vi "Test Customer Order Sent to Handler on Submit Order.vi"(8 "error in (no error)":errorcluster, 11 "Customer Test in":refnum<class "Customer Test.lvclass">=refnum) -> (0 "error out":errorcluster, 3 "Customer Test out":refnum<class "Customer Test.lvclass">)   [LabVIEW 2020, in "Customer Test.lvclass"]
uses:
  Customer Test.lvclass
  Processes/People/Customers/Customer/Customer.lvclass
  <vilib>/Astemes/Triarc Framework/Process/Process.lvclass
  Support/Beverages/TypeDefs/Options.ctl
  Support/Beverages/Beverage/Beverage.lvclass
  Support/Beverages/TypeDefs/Drink Type.ctl
  Test Doubles/Mock Job Handler/Mock Job Handler.lvclass
  C:/git/astemes-triarc-examples/source/Coffee Shop/Processes/People/Person/Person.lvclass
  C:/Program Files (x86)/National Instruments/LabVIEW 2020/vi.lib/Astemes/Triarc Framework/View/View.lvclass
  C:/Program Files (x86)/National Instruments/LabVIEW 2020/vi.lib/Astemes/Triarc Framework/Process/Process.lvclass
  C:/Program Files (x86)/National Instruments/LabVIEW 2020/vi.lib/Astemes/Triarc Framework/Base/Base.lvclass
  C:/Program Files (x86)/National Instruments/LabVIEW 2020/vi.lib/Astemes/Triarc Framework/Error Handler Interface/Error Handler Interface.lvclass
  C:/Program Files (x86)/National Instruments/LabVIEW 2020/vi.lib/Astemes/Triarc Framework/Logging/Logging.lvclass
  C:/git/astemes-triarc-examples/source/Coffee Shop/Processes/People/Customers/Customer/Customer.lvclass
  C:/git/astemes-triarc-examples/source/Coffee Shop/Processes/People/Process Job/Job Handler.lvclass
  C:/Program Files (x86)/National Instruments/LabVIEW 2020/vi.lib/Astemes/Triarc Framework/Async Handler/Async Handler.lvclass
  <vilib>/Astemes/LUnit/Test Case.lvclass
  C:/Program Files (x86)/National Instruments/LabVIEW 2020/vi.lib/Astemes/LUnit/Test Case.lvclass
  C:/Program Files (x86)/National Instruments/LabVIEW 2020/vi.lib/Astemes/LUnit/LUnit Runnable.lvclass
  C:/git/astemes-triarc-examples/source/Coffee Shop/Tests/Test Doubles/Mock Job Handler/Mock Job Handler.lvclass
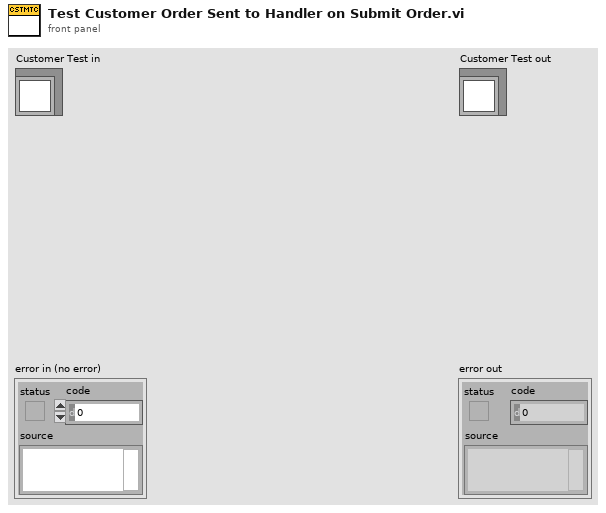
[diagram p1: front panel]
types:
  T1 = typedef "Beverage.lvclass/Drink Type.ctl" = enum16{"Dark Roast", "Decaf", "Espresso", "House Blend"}
  T2 = typedef "Beverage.lvclass/Options.ctl" = enum16{"<None>", "Milk", "Mocha", "Soy", "Whip"}
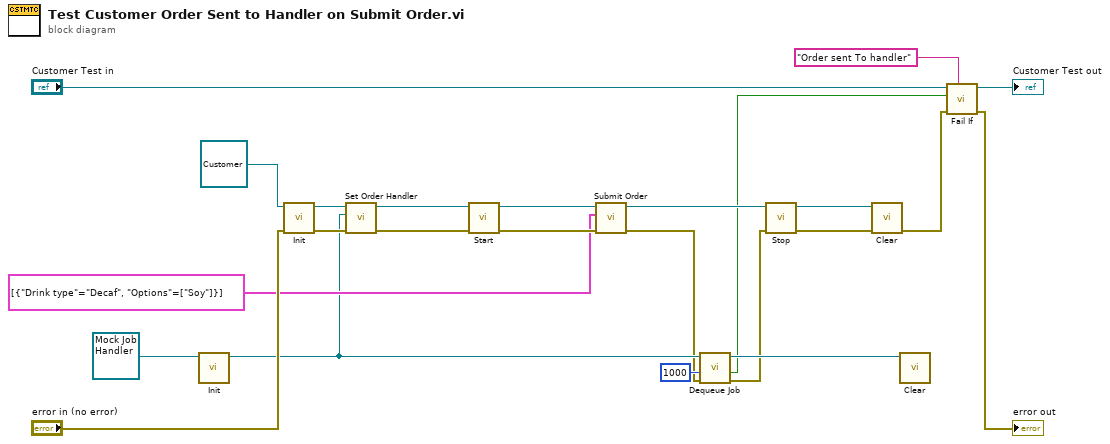
[diagram p0: block diagram]
diagram:
  n1 = call-dynamic "Init.vi"("Mock Job Handler In"=refnum<class "Mock Job Handler.lvclass"> refnum ("Mock Job Handler.lvclass")) -> ("Mock Job Handler Out"=w5:refnum<class "Mock Job Handler.lvclass">)  [unwired: 9 in, 1 out]
  n2 = call-dynamic "Init.vi"("error in (no error)"="error in (no error)", "View In"=refnum<class "Customer.lvclass"> refnum ("Customer.lvclass")) -> ("error out"=w23:errorcluster, "View Out"=w9:refnum<class "Customer.lvclass">)  [unwired: 8 in]
  n3 = call "Set Order Handler.vi"("error in (no error)"=w23, "Order Handler"=w5, "Customer In"=w9) -> ("error out"=w10:errorcluster, "Customer Out"=w8:refnum<class "Customer.lvclass">)  [unwired: 7 in]
  n4 = call <vilib>:"Start.vi"("error in (no error)"=w10, "Process In"=w8) -> ("error out"=w17:errorcluster, "Process Out"=w19:refnum<class "Customer.lvclass">)  [unwired: 7 in, 1 out]
  n5 = call "Submit Order.vi"("error in (no error)"=w17, "Order Content"=cluster{"Drink type":T1, "Options":T2[]}[] [{"Drink type"=enum."Decaf", "Options"=[enum."Soy"]}] ("Order"), "Customer In"=w19) -> ("error out"=w2:errorcluster, "Customer Out"=w18:refnum<class "Customer.lvclass">)  [unwired: 7 in]
  n6 = call "Dequeue Job.vi"("error in (no error)"=w2, "timeout in ms (-1)"=1000, "Mock Job Handler In"=w5) -> ("error out"=w1:errorcluster, "timed out?"=w3:bool, "Mock Job Handler Out"=w7:refnum<class "Mock Job Handler.lvclass">)  [unwired: 5 in, 1 out]
  n7 = call <vilib>:"Stop.vi"("error in (no error)"=w1, "Process In"=w18) -> ("error out"=w21:errorcluster, "Process Out"=w22:refnum<class "Customer.lvclass">)  [unwired: 7 in, 1 out]
  n8 = call-dynamic "Clear.vi"("error in (no error)"=w21, "View In"=w22) -> ("error out"=w14:errorcluster)  [unwired: 9 in]
  n9 = call-dynamic "Clear.vi"("Mock Job Handler In"=w7) -> ()  [unwired: 10 in, 1 out]
  n10 = call <vilib>:"Fail If.vi"("Description"="Order sent To handler", "error in (no error)"=w14, "Fail?"=w3, "LUnit Test Case In"="Customer Test in") -> ("error out"=→"error out":errorcluster, "LUnit Test Case Out"=→"Customer Test out":refnum<class "Test Case.lvclass">)  [unwired: 6 in]
